vi "target selector.vi"() -> (1 "Canceled?":bool, 3 "Target Index":i32)   [LabVIEW 2013]
panel:
  in  "Cancel":bool
  in  "OK":bool
  in  "Select Target":enum16{"Tanner", "cRIO", "PC"}(ring)
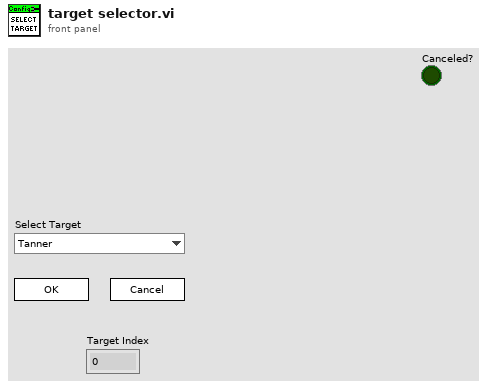
[diagram p1: front panel]
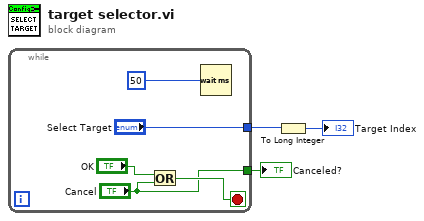
[diagram p0: block diagram]
diagram:
  n1 = while {
    tunnel: ["Select Target"] -> w2
    tunnel: ["Cancel"] -> w3
    stop <- w5 stop-if-true
    n2 = Or(x="OK", y="Cancel") -> (x .or. y?=w5:bool)
    n3 = Wait (ms)(milliseconds to wait=u32 50) -> ()  [unwired: 1 out]
  }
  "Canceled?" <- w3
  n4 = To Long Integer(number=w2) -> (32bit integer=→"Target Index":i32)
